vi "Sort.vi"() -> ()   [LabVIEW 2015]
panel:
  in  "Space size":i32=5000
  in  "prod":i32=8
  in  "sort":i32=8
  in  "stop":bool
  out "size(s)":i32
  out "data":u32[](array[numeric])
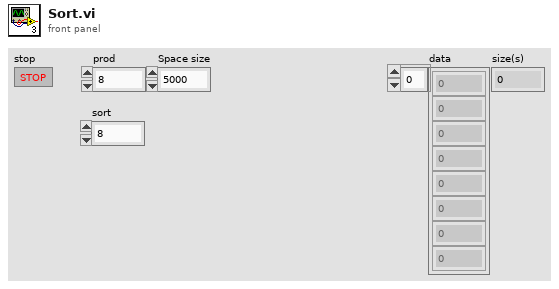
[diagram p1: front panel]
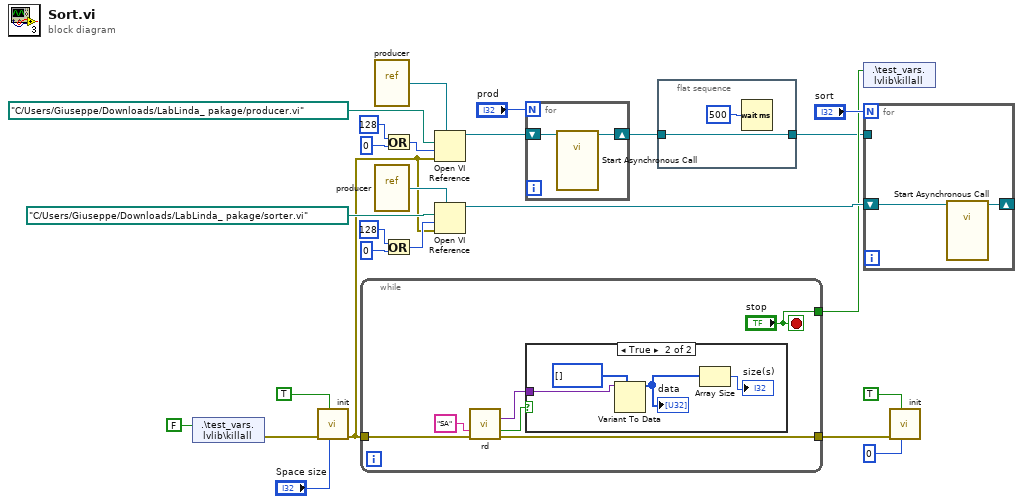
[diagram p0: block diagram]
diagram:
  n1 = shared-variable ".\\test_vars.lvlib\\killall"(FALSE ("killall")) -> (error out=w3:errorcluster)  [unwired: 1 in]
  n2 = call "init.vi"("Space size"="Space size", "Cleaneup"=TRUE, "error in (no error)"=w3) -> ("error out"=w10:errorcluster)  [unwired: 8 in]
  n3 = while {
    tunnel: w10 -> [w28]
    tunnel: [w27] -> w9
    tunnel: ["stop"] -> w5
    stop <- "stop" stop-if-true
    n4 = call "rd.vi"("Name in"="SA", "error in (no error)"=w28) -> ("OUT VARIANT"=w30:variant, "Valid data"=w29:bool, "error out"=w27:errorcluster)  [unwired: 11 in]
    n5 = case shown="True" w29 {
      tunnel: w30 -> [_ w34]
      frame False {
      }
      frame True {
        n6 = Variant To Data(type=u32[] [], Variant=w34) -> (data=w33:u32[])  [unwired: 1 in, 1 out]
        "data" <- w33
        n7 = Array Size(array=w33) -> (size(s)=→"size(s)":i32)
      }
    }
  }
  n8 = vi-ref "producer.vi"() -> (w25:refnum<vi>)
  n9 = vi-ref "producer.vi"() -> (w12:refnum<vi>)
  n10 = Or(x=128 ("options"), y=0) -> (x .or. y?=w21:i32)
  n11 = Or(x=128 ("options"), y=0) -> (x .or. y?=w16:i32)
  n12 = Open VI Reference(type specifier VI Refnum (for type only)=w25, vi path=path "C:/Users/Giuseppe/Downloads/LabLinda_ pakage/producer.vi", options=w21, error in (no error)=w10) -> (vi reference=w20:refnum<vi>)  [unwired: 2 in, 1 out]
  n13 = Open VI Reference(type specifier VI Refnum (for type only)=w12, vi path=path "C:/Users/Giuseppe/Downloads/LabLinda_ pakage/sorter.vi", options=w16, error in (no error)=w10) -> (vi reference=w17:refnum<vi>)  [unwired: 2 in, 1 out]
  n14 = for {
    N: "prod" -> [_]
    shift-right: [w36] -> w2
    shift-left: w20 -> [w37]
    n15 = call-by-ref "Start Asynchronous Call"(reference=w37) -> (reference out=w36:refnum<vi>)  [unwired: 13 in, 1 out]
  }
  n16 = flat-sequence {
    tunnel: w2 -> [w39]
    tunnel: [w39] -> w1
    frame #0 {
      n17 = Wait (ms)(milliseconds to wait=u32 500) -> ()  [unwired: 1 out]
    }
  }
  n18 = shared-variable ".\\test_vars.lvlib\\killall"(w5) -> ()  [unwired: 1 in, 1 out]
  n19 = for {
    N: "sort" -> [_]
    shift-right: [w40] -> _
    shift-left: w17 -> [w41]
    tunnel: w1 -> [_]
    n20 = call-by-ref "Start Asynchronous Call"(reference=w41) -> (reference out=w40:refnum<vi>)  [unwired: 13 in, 1 out]
  }
  n21 = call "init.vi"("Space size"=0, "Cleaneup"=TRUE, "error in (no error)"=w9) -> ()  [unwired: 8 in, 1 out]
